vi "Enable Sync Mask.vi"(8 "error in (no error)":errorcluster, 10 "Enable":bool, 11 "Scheduler in":refnum<class "Scheduler.lvclass">=refnum) -> (0 "error out":errorcluster, 3 "Scheduler out":refnum<class "Scheduler.lvclass">)   [LabVIEW 2020, in "CIRCUS_uServices.lvlib" / "Holy Trinity.lvlib" / "Scheduler.lvlib" / "Scheduler.lvclass"]
doc: "VI for change control state between 'enabled' and 'disabled and grayed out.' This VI also resets the values in the mask whenever it is disabled."
uses:
  Scheduler.lvclass
  TALOS/TALOS_PPL.lvlibp/Father of all uServices/Father of all uServices/Father of all uServices.lvclass
  TALOS/TALOS_PPL.lvlibp
  C:/Users/marco/Documents/GitHub_Lab/CIRCUS/TALOS/TALOS_PPL.lvlibp/Ancestor/Ancestor/Ancestor.lvclass
  C:/Users/marco/Documents/GitHub_Lab/CIRCUS/TALOS/Actor Framework.lvlibp/1abvi3w/vi.lib/ActorFramework/Actor/Actor.lvclass
  C:/Users/marco/Documents/GitHub_Lab/CIRCUS/TALOS/TALOS_PPL.lvlibp/Father of all uServices/Father of all uServices/Father of all uServices.lvclass
  Run Utilities/TypeDefs/Synchronize FPGA Cluster.ctl
  Run Utilities/Run Utilities.lvlib
panel:
  in  "Sync. mask - template":T1[](array[typedef])
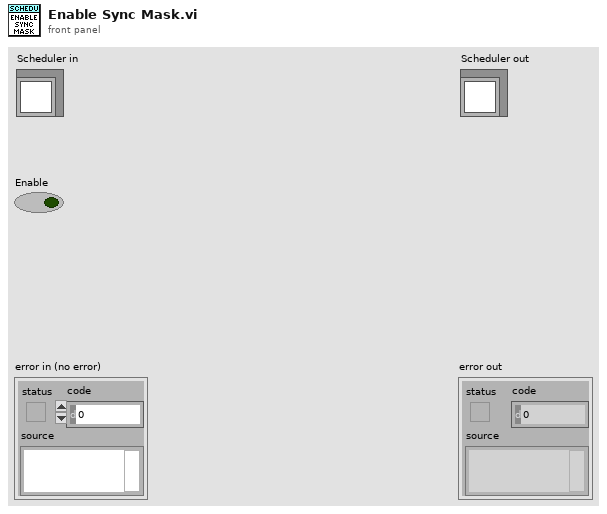
[diagram p1: front panel]
types:
  T1 = typedef "CIRCUS_uServices.lvlib/Run Utilities.lvlib/Synchronize FPGA Cluster.ctl" = cluster{"Status":bool, "FPGA Name":string}
  T2 = enum8{"Enabled", "Disabled", "Disabled and Grayed Out"}
  T3 = typedef "TALOS.lvlib/Run Utilities.lvlib/Synchronize Kasli Cluster.ctl" = cluster{"Status":bool, "FPGA Name":string}
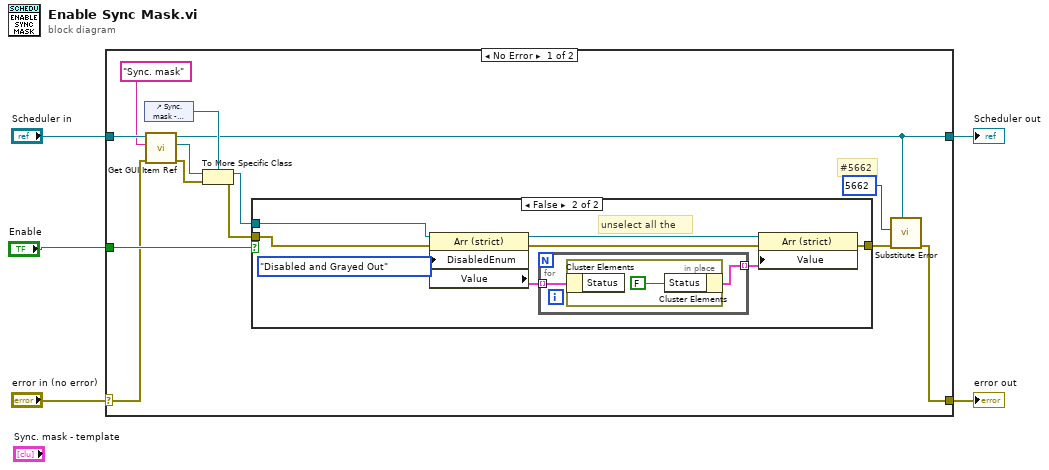
[diagram p0: block diagram]
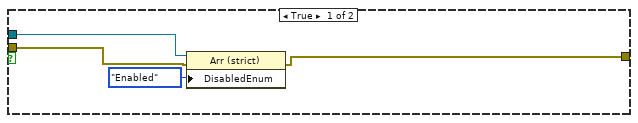
[diagram p2: hidden frame]
diagram:
  n1 = case shown="No Error" "error in (no error)" {
    selector: "error in (no error)" -> [w15 w35]
    tunnel: [w8 w35] -> w4
    tunnel: [w7 w34] -> w2
    tunnel: "Scheduler in" -> [w17 w34]
    tunnel: "Enable" -> [w18 _]
    frame No Error {
      # "#5662"
      n2 = control-ref of="Sync. mask - template"() -> (w10:refnum<vi>)
      n3 = call "Get GUI Item Ref.vi"("error in (no error)"=w15, "FP Item Name"="Sync. mask", "uService Template in"=w17) -> ("error out"=w12:errorcluster, "Ctl Refnum"=w14:refnum<vi>, "uService Template out"=w7:refnum<class "Father of all uServices.lvclass">)  [unwired: 6 in]
      n4 = To More Specific Class(target class=w10, reference=w14, error in=w12) -> (specific class reference=w13:refnum<vi>, error out=w11:errorcluster)
      n5 = case shown="False" w18 {
        tunnel: w13 -> [w21 w24]
        tunnel: w11 -> [w19 w26]
        tunnel: [w20 w23] -> w9
        frame True {
          n6 = property class="Arr (strict)"(reference=w21, error in=w19, "DisabledEnum"=T2."Enabled" ("Disabled")) -> (error out=w20:errorcluster)  [unwired: 1 out]
        }
        frame False {
          # "unselect all the"
          n7 = property class="Arr (strict)"(reference=w24, error in=w26, "DisabledEnum"=T2."Disabled and Grayed Out" ("Disabled")) -> (reference out=w27:refnum<vi>, error out=w25:errorcluster, "Value"=w29:T3[])
          n8 = for {
            tunnel: w29 -> [w32] mode=indexing
            tunnel: [w31] -> w28 mode=indexing
            n9 = in-place {
              n10 = in-place-cluster #1(w32) -> ()  [unwired: 1 out]
              n11 = in-place-cluster #1("Status"=FALSE) -> (w31:T3)
            }
          }
          n12 = property class="Arr (strict)"(reference=w27, error in=w25, "Value"=w28) -> (error out=w23:errorcluster)  [unwired: 1 out]
        }
      }
      n13 = call "Substitute Error.vi"("LabVIEW Object"=w7, "error in (no error)"=w9, "Error Code"=5662) -> ("error out"=w8:errorcluster)  [unwired: 8 in]
    }
    frame Error {
    }
  }
  "error out" <- w4
  "Scheduler out" <- w2
